vi "Register Call.vi"(8 "error in (no error)":errorcluster, 11 "LabSpy":refnum<data-value>) -> (0 "error out":errorcluster, 3 "LabSpy Out":refnum<data-value>)   [LabVIEW 2013, in "LabSpy.lvclass"]
uses:
  LabSpy.lvclass
  LabSpy.lvclass/LabSpy.ctl
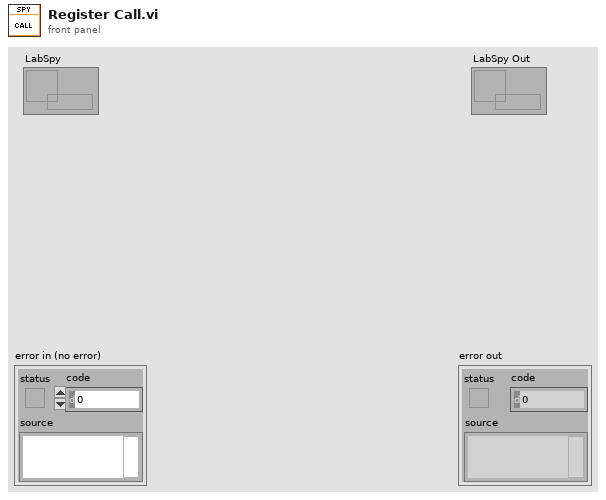
[diagram p1: front panel]
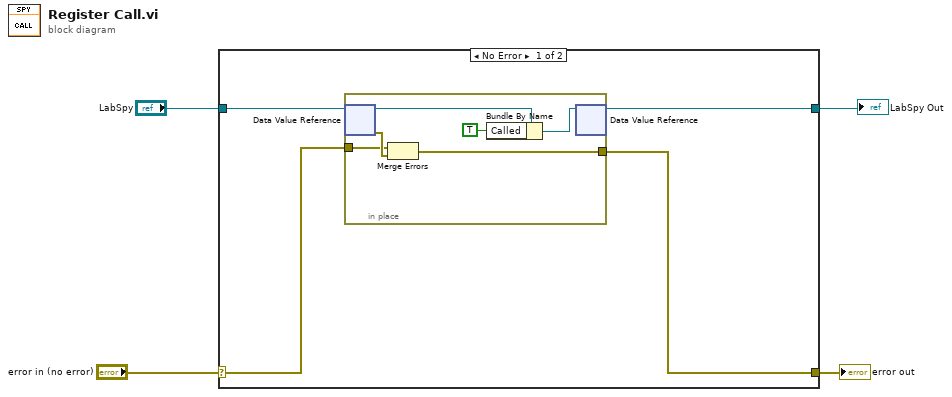
[diagram p0: block diagram]
diagram:
  n1 = case shown="No Error" "error in (no error)" {
    selector: "error in (no error)" -> [w6 w16]
    tunnel: [w5 w16] -> w3
    tunnel: [w7 w15] -> w1
    tunnel: "LabSpy" -> [w8 w15]
    frame No Error {
      n2 = in-place {
        in-place-border: w6 -> [w10]
        in-place-border: [w9] -> w5
        n3 = in-place-dvr #1(w8) -> (w14:refnum<class "LabSpy.lvclass">, w11:errorcluster)
        n4 = Merge Errors(w10, w11) -> (w9:errorcluster)
        n5 = Bundle By Name(cluster=w14, "Called"=TRUE) -> (w13:refnum<class "LabSpy.lvclass">)
        n6 = in-place-dvr #1(w13) -> (w7:refnum<data-value>)  [unwired: 1 out]
      }
    }
    frame Error {
    }
  }
  "error out" <- w3
  "LabSpy Out" <- w1
